vi "Obtain Notifiers.vi"(8 "error in (no error)":errorcluster, 11 "PID Loop in":refnum<class "PID Loop.lvclass">) -> (0 "error out":errorcluster, 3 "PID Loop out":refnum<class "PID Loop.lvclass">)   [LabVIEW 2024, in "PID Loop.lvlib" / "PID Loop.lvclass"]
uses:
  PID Loop.lvclass
  PID Loop.lvclass/PID Loop.ctl
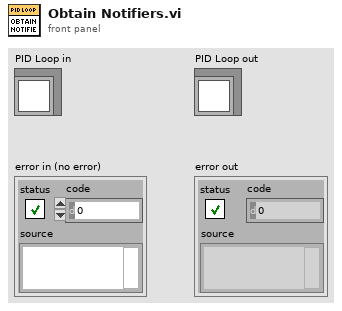
[diagram p1: front panel]
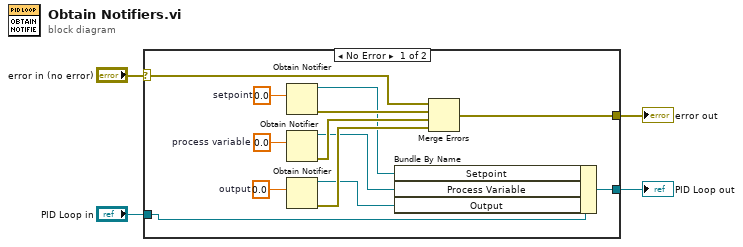
[diagram p0: block diagram]
diagram:
  n1 = case shown="No Error" "error in (no error)" {
    selector: "error in (no error)" -> [w5 w19]
    tunnel: [w10 w19] -> w3
    tunnel: [w9 w18] -> w1
    tunnel: "PID Loop in" -> [w11 w18]
    frame No Error {
      w12 = 0.0  # output
      w13 = 0.0  # process variable
      w14 = 0.0  # setpoint
      n2 = Obtain Notifier(notification data type=w14) -> (notifier out=w8:refnum<notifier>, error out=w17:errorcluster)  [unwired: 3 in, 1 out]
      n3 = Obtain Notifier(notification data type=w13) -> (notifier out=w7:refnum<notifier>, error out=w16:errorcluster)  [unwired: 3 in, 1 out]
      n4 = Obtain Notifier(notification data type=w12) -> (notifier out=w6:refnum<notifier>, error out=w15:errorcluster)  [unwired: 3 in, 1 out]
      n5 = Bundle By Name(cluster=w11, "Setpoint"=w8, "Process Variable"=w7, "Output"=w6) -> (w9:refnum<class "PID Loop.lvclass">)
      n6 = Merge Errors(w5, w17, w16, w15) -> (w10:errorcluster)
    }
    frame Error {
    }
  }
  "error out" <- w3
  "PID Loop out" <- w1
